vi "DIVIDI TRASDUTTORI PER TIPO.vi"(11 "all rows":string[][](array[string])) -> (3 "PAGINE TRASDUTTORI":string[][][](array[string]))   [LabVIEW 2019]
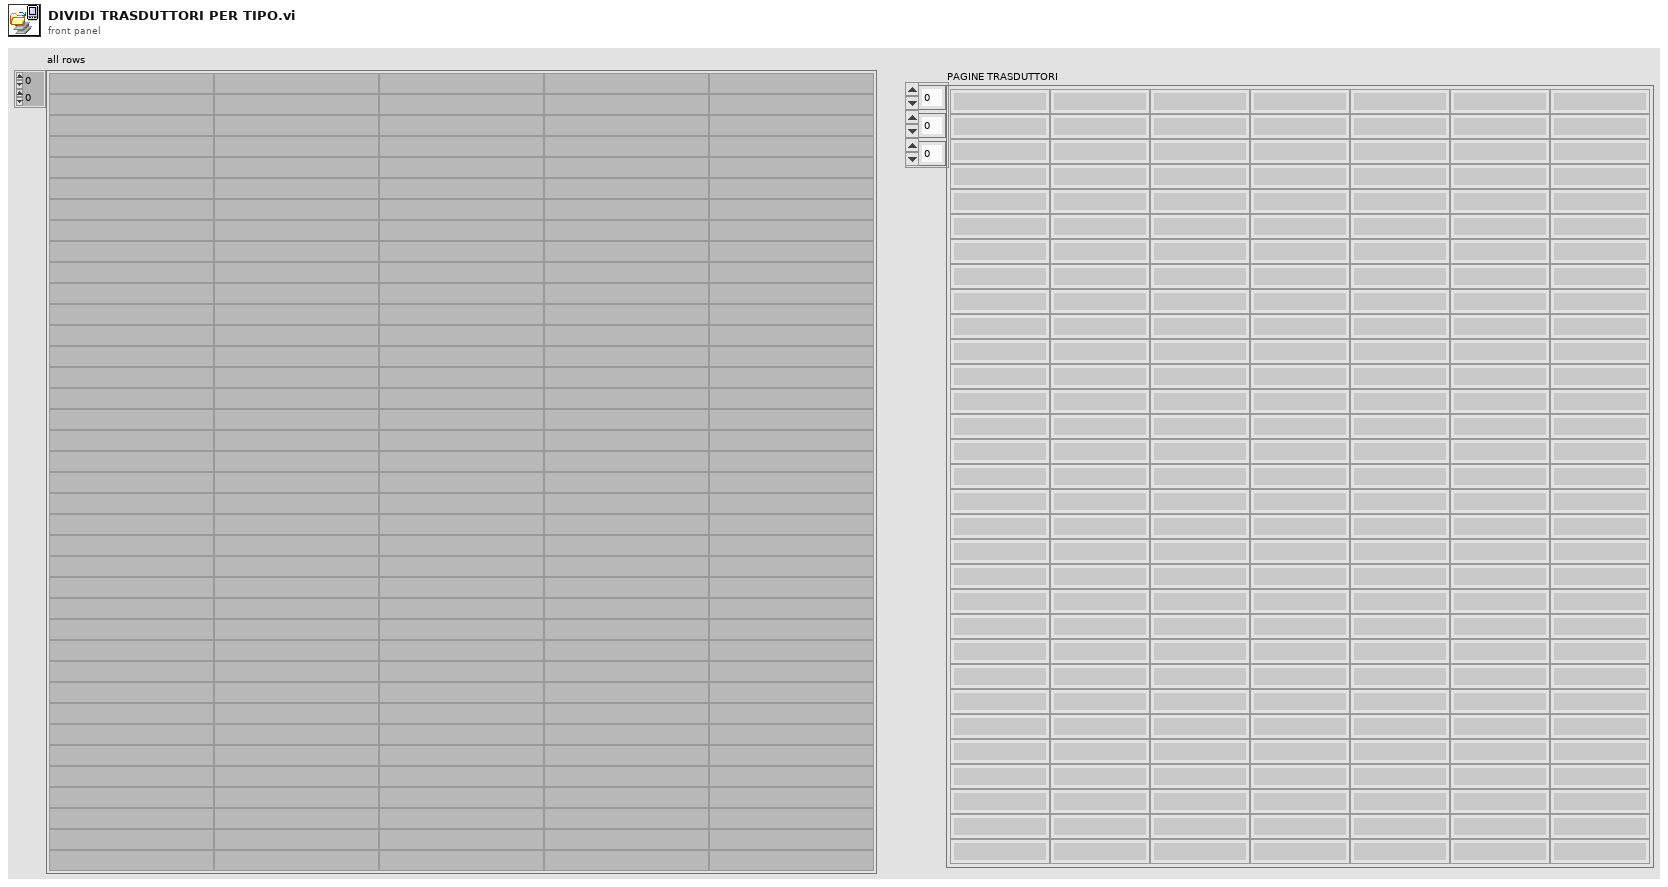
[diagram p1: front panel]
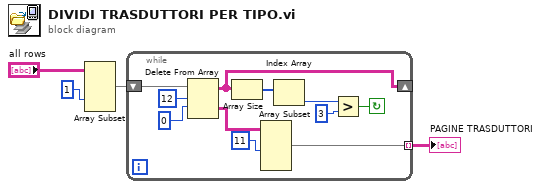
[diagram p0: block diagram]
diagram:
  n1 = Array Subset(array="all rows", index (col)=1 ("index")) -> (w1:string[][])  [unwired: 3 in]
  n2 = while {
    shift-right: [w9] -> _
    shift-left: w1 -> [w15]
    tunnel: [w10] -> w4 mode=indexing
    stop <- w5 continue-if-true
    n3 = Delete From Array(array=w15, length=12, index (row)=0) -> (deleted portion=w12:string[][], array with subset deleted=w9:string[][])  [unwired: 1 in]
    n4 = Array Size(array=w9) -> (size(s)=w8:i32[])
    n5 = Array Subset(array=w12, length (row)=11 ("length")) -> (w10:string[][])  [unwired: 3 in]
    n6 = Index Array(array=w8) -> (element=w7:i32)  [unwired: 1 in]
    n7 = Greater?(x=w7, y=3) -> (0:w5:bool)
  }
  "PAGINE TRASDUTTORI" <- w4
